vi "Endpoint ID.vi"(10 "Remote Port":u16, 11 "Remote Address":string) -> (3 "Endpoint ID":string)   [LabVIEW 2020, in "Vecto.lvlib" / "TCPMessaging.lvclass"]
uses:
  TCPMessaging.lvclass
  TCPMessaging.lvclass/TCPMessaging.ctl
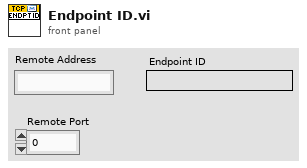
[diagram p1: front panel]
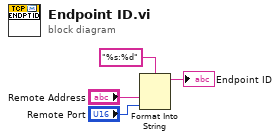
[diagram p0: block diagram]
diagram:
  n1 = Format Into String(format string="%s:%d", "Remote Address", "Remote Port") -> (resulting string=→"Endpoint ID":string)  [unwired: 2 in, 1 out]
